vi "Lockin Channel Logic.vi"(10 "Old Channels":T1, 11 "New Channels":T1) -> (2 "index of element":i32, 3 "Channels Out":T1)   [LabVIEW 2020]
uses:
  Lockin Channels.ctl
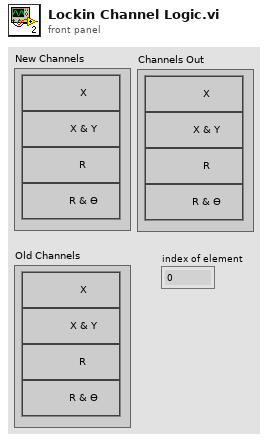
[diagram p1: front panel]
types:
  T1 = typedef "Lockin Channels.ctl" = cluster{"X":bool, "X&Y":bool, "R":bool, "R & ϴ":bool}
  T2 = cluster{"Old Channels[0]":bool, "Old Channels[1]":bool, "Old Channels[2]":bool, "Old Channels[3]":bool}
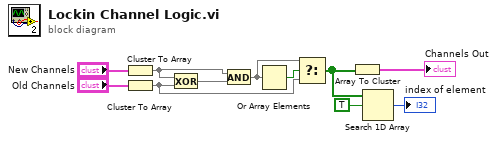
[diagram p0: block diagram]
diagram:
  n1 = Cluster To Array(cluster="New Channels") -> (array=w2:bool[])
  n2 = Cluster To Array(cluster="Old Channels") -> (array=w9:bool[])
  n3 = Exclusive Or(1:w9, 2:w2) -> (0:w1:bool[])
  n4 = And(x=w2, y=w1) -> (x .and. y?=w7:bool[])
  n5 = Or Array Elements(Boolean array=w7) -> (logical OR=w6:bool)
  n6 = Select(t=w7, s=w6, f=w9) -> (s? t:f=w8:bool[])
  n7 = Array To Cluster(array=w8) -> (cluster=→"Channels Out":T2)
  n8 = Search 1D Array(1D array=w8, element=TRUE) -> (index of element=→"index of element":i32)  [unwired: 1 in]
